vi "ExperimentStateSave.vi"(0 "Experiment State":T1={"error"={"status"=FALSE, "code"=0, "source"=""}, "Digitizer DAQmx Tasks"={"TaskArray"=[]}, "Digitizer Settings"={"Channel Settings"=[], "Card Settings"=[]}, "Synchronization Settings"={"Synchronizer"="PXI1Slot2", "source terminal"="GlobalSoftwareTrigger"}, "Digitizer Data"=[], "Next Shot#"="0", "System Message"="", "User Shot Notes"="", "Timing Settings"={"Timing Card Settings"=[], "Timing Channel Settings"=[[{"Delay (s)"=2.559999942779541, "Pulse width (s)"=0.009999999776482582, "Active"=TRUE, "Channel Name"="Fiber 8", "counter"="PXI1Slot8/ctr7"}]]}, "Timing Tasks"={"TaskArray"=[]}, "Tree"="0"} {"Timing Settings"."Timing Channel Settings"."Pulse width (s)" format="%.3p"; "Timing Settings"."Timing Channel Settings"."Delay (s)" format="%.3p"; "Digitizer Settings"."Card Settings"."Global Edge Type" items=["Rising"=10280, "Falling"=10171]; "Digitizer Settings"."Card Settings"."Sample Rate" format="%#_3p"}, 2 "Shot Quality":string(combo), 3 "Error In":errorcluster, 4 "Tree Path":string="proto_tree") -> (6 "Error Message":errorcluster)   [LabVIEW 2013]
uses:
  Controls/ExperimentStateCluster.ctl
  Controls/DigitizerSettingsChannelSettings.ctl
  Controls/DigitizerSettingsCardSettingsArray.ctl
  Controls/DigitizerSettingsCardSettings.ctl
  Controls/TimingCardSettings.ctl
  Controls/TimingChannelSettings.ctl
  <vilib>/MDSplus/Library/MDSplus.lvlib
  <vilib>/MDSplus/Classes/Tree_Class/Tree.lvclass
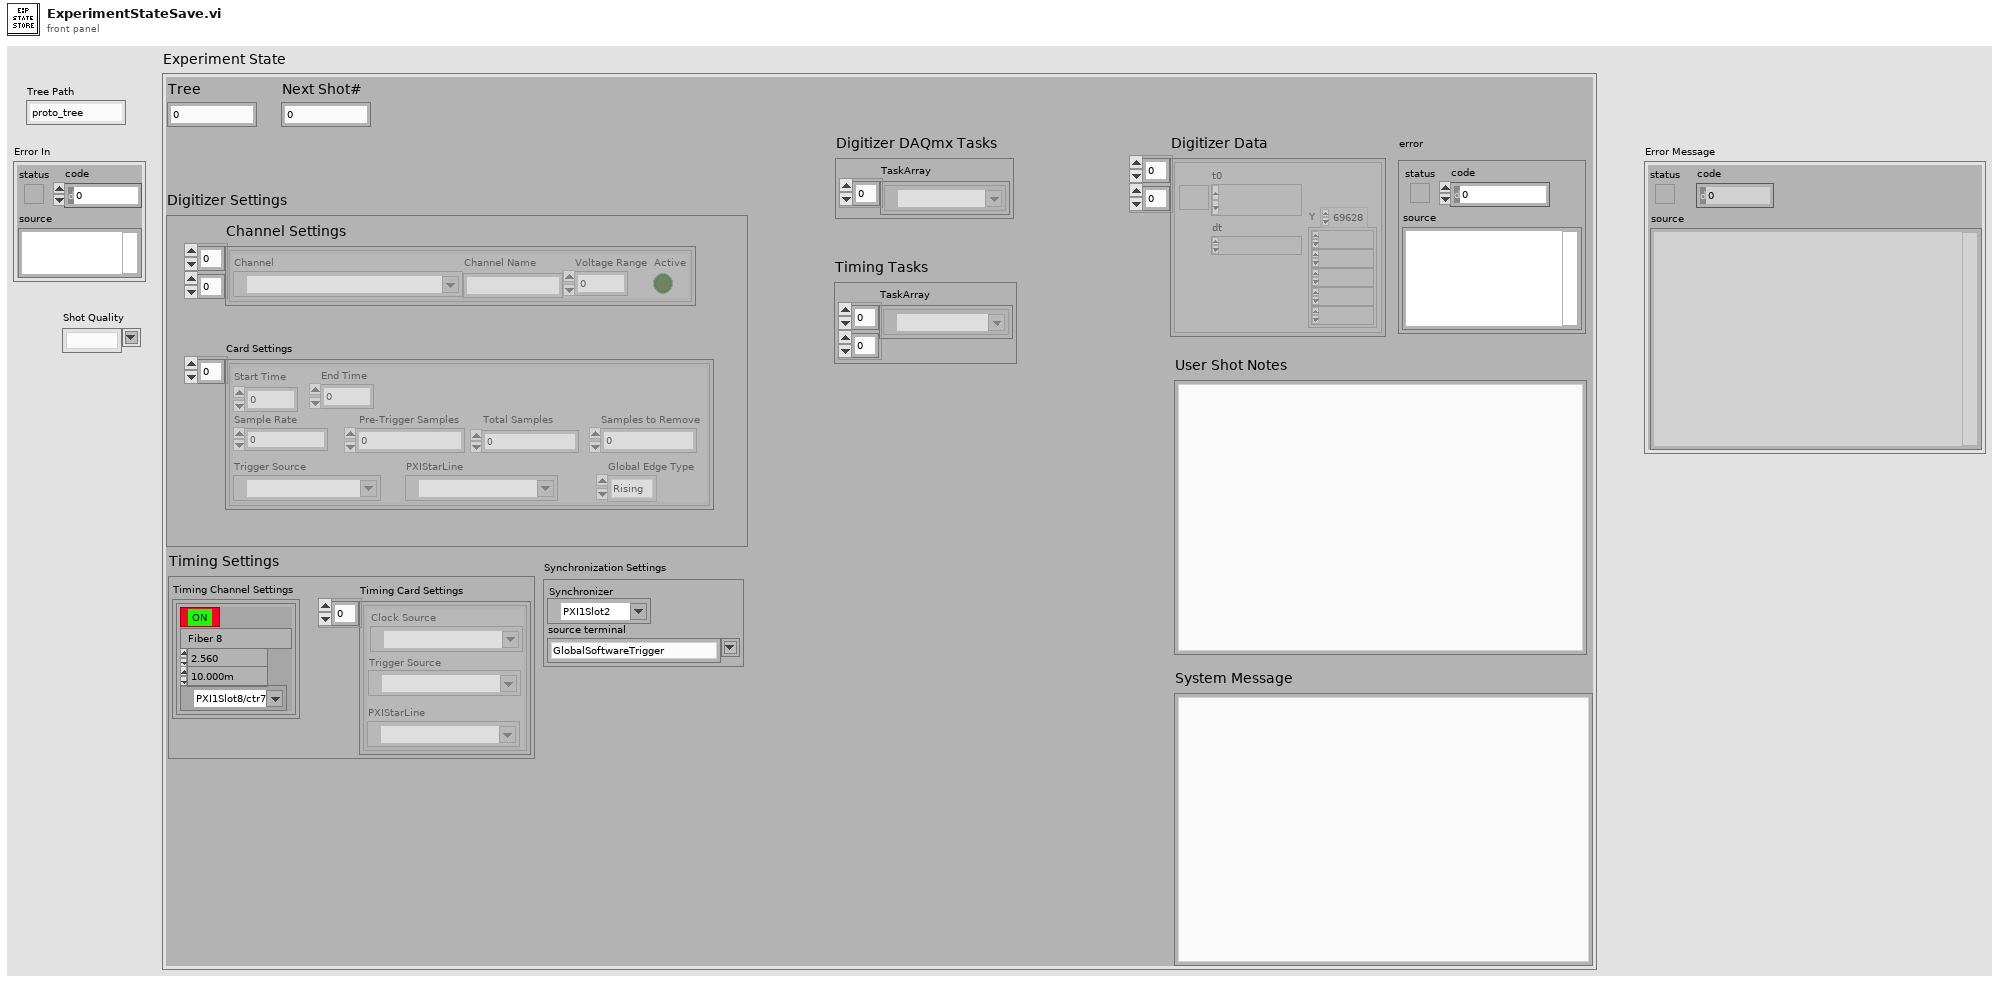
[diagram p1: front panel]
types:
  T1 = typedef "ExperimentStateCluster.ctl" = cluster{"error":errorcluster, "Digitizer DAQmx Tasks":cluster{"TaskArray":refnum<k21>[]}, "Digitizer Settings":cluster{"Channel Settings":T2[][], "Card Settings":T3}, "Synchronization Settings":cluster{"Synchronizer":refnum<k15>, "source terminal":string}, "Digitizer Data":waveform(dbl)[][], "Next Shot#":string, "System Message":string, "User Shot Notes":string, "Timing Settings":cluster{"Timing Card Settings":T5[], "Timing Channel Settings":T6[][]}, "Timing Tasks":cluster{"TaskArray":refnum<k21>[][]}, "Tree":string}
  T2 = typedef "DigitizerSettingsChannelSettings.ctl" = cluster{"Channel":tag, "Channel Name":string, "Voltage Range":dbl, "Active":bool}
  T3 = typedef "DigitizerSettingsCardSettingsArray.ctl" = T4[]
  T4 = typedef "DigitizerSettingsCardSettings.ctl" = cluster{"Start Time":dbl, "End Time":dbl, "Sample Rate":dbl, " Pre-Trigger Samples":u32, "Total Samples":i32, "Samples to Remove":u32, "Trigger Source":tag, "Global Edge Type":i32, "PXIStarLine":tag}
  T5 = typedef "TimingCardSettings.ctl" = cluster{"Trigger Source":tag, "Clock Source":tag, "PXIStarLine":tag}
  T6 = typedef "TimingChannelSettings.ctl" = cluster{"Delay (s)":dbl, "Pulse width (s)":dbl, "Active":bool, "Channel Name":string, "counter":tag}
  T7 = cluster{"Channel Settings":T2[][], "Card Settings":T3}
  T8 = cluster{"Timing Card Settings":T5[], "Timing Channel Settings":T6[][]}
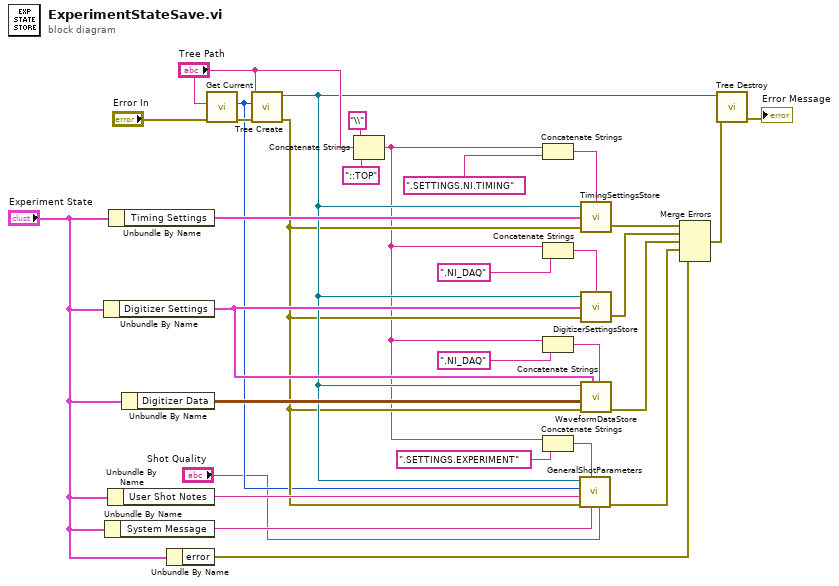
[diagram p0: block diagram]
diagram:
  n1 = Unbundle By Name("Experiment State") -> ("Digitizer Settings"=w12:T7)
  n2 = Unbundle By Name("Experiment State") -> ("System Message"=w18:string)
  n3 = Unbundle By Name("Experiment State") -> ("User Shot Notes"=w19:string)
  n4 = Unbundle By Name("Experiment State") -> ("Timing Settings"=w20:T8)
  n5 = Unbundle By Name("Experiment State") -> ("Digitizer Data"=w13:waveform(dbl)[][])
  n6 = Unbundle By Name("Experiment State") -> ("error"=w7:errorcluster)
  n7 = call <vilib>:"Get Current.vi"("error in (no error)"="Error In", "Tree name"="Tree Path") -> ("error out"=w31:errorcluster, "Current shot out"=w9:i32)  [unwired: 7 in, 1 out]
  n8 = call <vilib>:"Tree Create.vi"("error in (no error)"=w31, "Shot"=w9, "Name"="Tree Path") -> ("error out"=w10:errorcluster, "Tree DVR out"=w11:refnum<data-value>)  [unwired: 7 in]
  n9 = Concatenate Strings("\\" ("string"), "Tree Path", "::TOP" ("string")) -> (w6:string)
  n10 = Concatenate Strings(w6, ".SETTINGS.NI.TIMING" ("string")) -> (w21:string)
  n11 = Concatenate Strings(w6, ".NI_DAQ" ("string")) -> (w23:string)
  n12 = Concatenate Strings(w6, ".NI_DAQ") -> (w17:string)
  n13 = Concatenate Strings(w6, ".SETTINGS.EXPERIMENT" ("string")) -> (w4:string)
  n14 = call "GeneralShotParameters.vi"("Shot Quality"="Shot Quality", "System Message"=w18, "TreeNode Path In"=w4, "Error In"=w10, "User Shot Notes"=w19, "Current shot"=w9, "Tree DVR Input"=w11) -> ("Error Out"=w8:errorcluster)  [unwired: 4 in]
  n15 = call "TimingSettingsStore.vi"("Tree Path In"=w21, "error in"=w10, "Timing Settings"=w20, "Tree DVR In"=w11) -> ("error out"=w15:errorcluster)  [unwired: 1 in]
  n16 = call "DigitizerSettingsStore.vi"("Tree Path In"=w23, "error in"=w10, "Digitizer Settings"=w12, "Tree DVR In"=w11) -> ("error out"=w14:errorcluster)  [unwired: 1 in]
  n17 = call "WaveformDataStore.vi"("Digitizer Settings"=w12, "error in"=w10, "Digitizer Data"=w13, "Tree Path In"=w17, "Tree DVR In"=w11) -> ("error out"=w16:errorcluster)  [unwired: 6 in]
  n18 = Merge Errors(w15, w14, w16, w8, w7) -> (w29:errorcluster)
  n19 = call <vilib>:"Tree Destroy.vi"("error in (no error)"=w29, "Tree DVR in"=w11) -> ("error out"=→"Error Message":errorcluster)  [unwired: 9 in]
